vi "Front Panel Key Press.vi"(8 "error in (no error)":errorcluster, 10 "Front Panel Key":T1(ring), 11 "VISA resource name":refnum<visa-resource-name>) -> (0 "error out":errorcluster, 3 "VISA resource name out":refnum<visa-resource-name>)   [LabVIEW 2009, in "SR400.lvlib"]
doc: "The CK command simulates pressing a front panel\nkey. j is a required parameter from 0 to 13. The\nCK command may be sent at any time and is not\nrestricted by the remote/local state of the front\npanel.\nj key\n0 DOWN CURSOR\n1 RIGHT CURSOR\n2 LEVEL\n3 SETUP\n4 COM\n5 STOP\n6 LOCAL\n7 RESET\n8 LEFT CURSOR\n9 UP CURSOR\n10 MODE\n11 AGATE\n12 BGATE\n13 START"
uses:
  SR400.lvlib
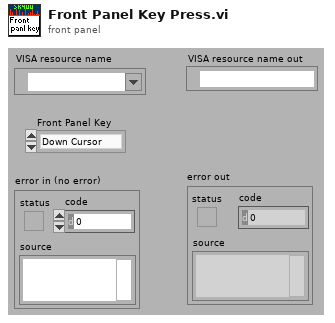
[diagram p1: front panel]
types:
  T1 = enum16{"Down Cursor", "Right Cursor", "Level", "Setup", "Com", "Stop", "Local", "Reset", "Left Cursor", "Up Cursor", "Mode", "A Gate", "B Gate", "Start"}
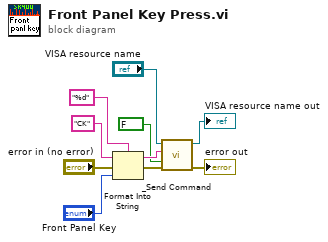
[diagram p0: block diagram]
diagram:
  n1 = Format Into String(format string="%d", initial string="CK" ("command"), error in="error in (no error)", "Front Panel Key") -> (resulting string=w5:string, error out=w4:errorcluster)
  n2 = call "_Send Command.vi"("error in (no error)"=w4, "Query? (F)"=FALSE, "Command"=w5, "VISA resource name"="VISA resource name") -> ("error out"=→"error out":errorcluster, "VISA resource name out"=→"VISA resource name out":refnum<visa-resource-name>)  [unwired: 6 out]
